vi "mock resonant image1.vi"() -> (0 "samples per period (var pix clock)":i32, 2 "var dwell time in ticks (2*pi)":i32[](graph) caption="dwell time in ticks (2*pi)", 3 "var dwell time in ticks (pi/2)":i16[](graph) caption="dwell time in ticks (pi/2)", 4 "samples per period (fix pix clock)":i32, 6 "fixed dwell time":i32)   [LabVIEW 2012]
uses:
  <vilib>/Analysis/NI_AALBase.lvlib
panel:
  out "avg dwell time":dbl
  out "x/y":dbl
  out "sum":i32
  out "cumsum 2":i32[](graph)
  in  "two lines per cycle":i32=2
  out "size(s)":i32
  out "samples per line":dbl
  out "cumsum":i32[](graph)
  out "Histogram Graph":T1(graph)
  in  "x pixels":i32=780
  out "Waveform Graph":dbl[](graph)
  out "Image":T2(plugin-control)
  in  "lines in y":i32=1
  in  "resonant frequency (eg. 8kHz)":i32=8000
  in  "sample clock (eg. 40 MHz)":i32=40000000
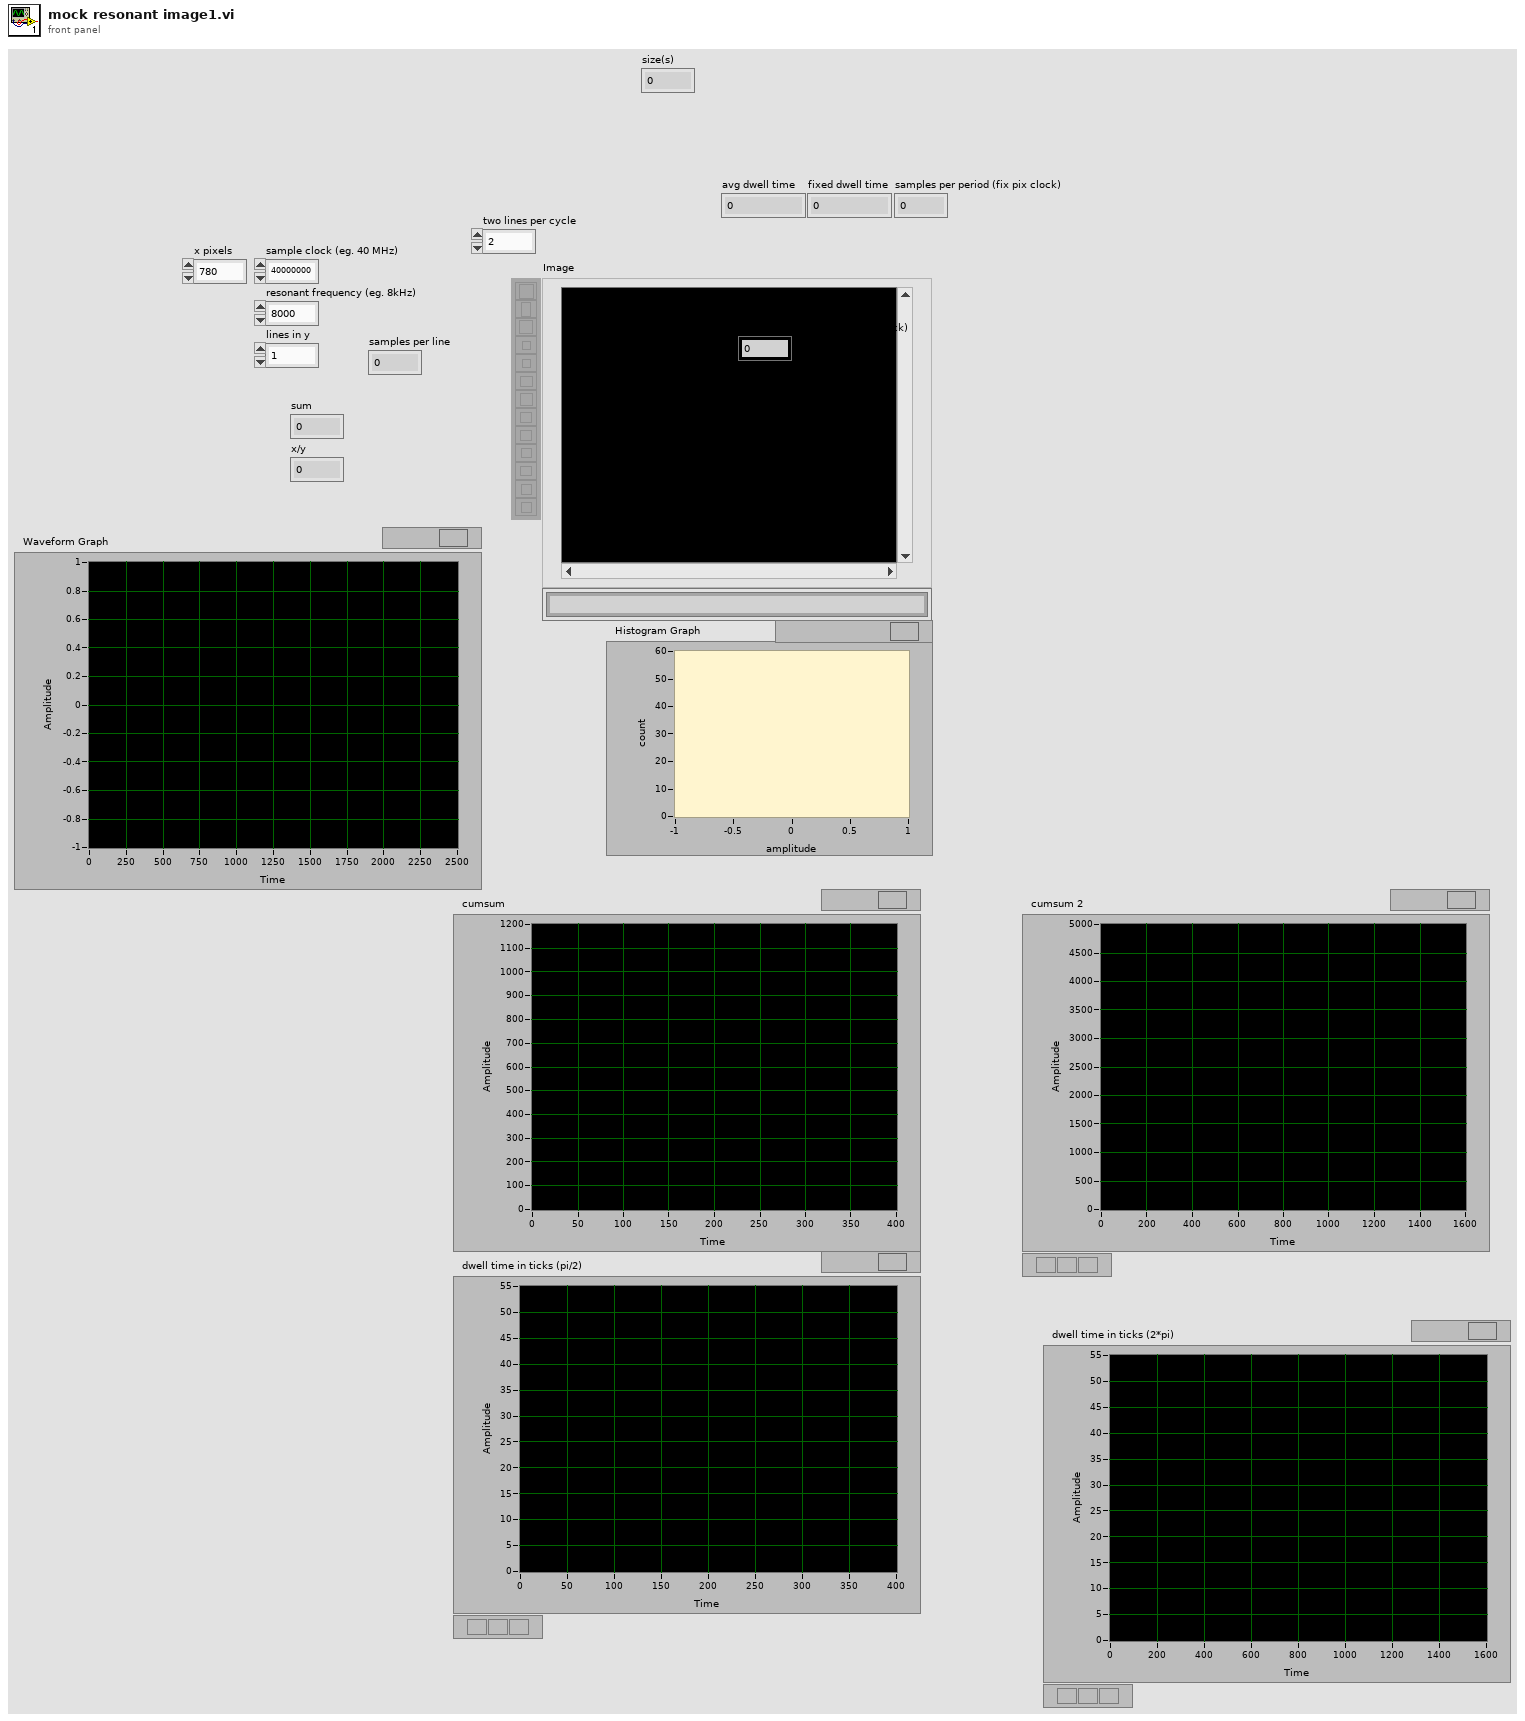
[diagram p1: front panel]
types:
  T1 = cluster{"X Values":dbl[], "Histogram: h(x)":i32[]}
  T2 = typedef "IMAQ Image.ctl" = refnum<image>
  T3 = typedef "Image Type" = u32
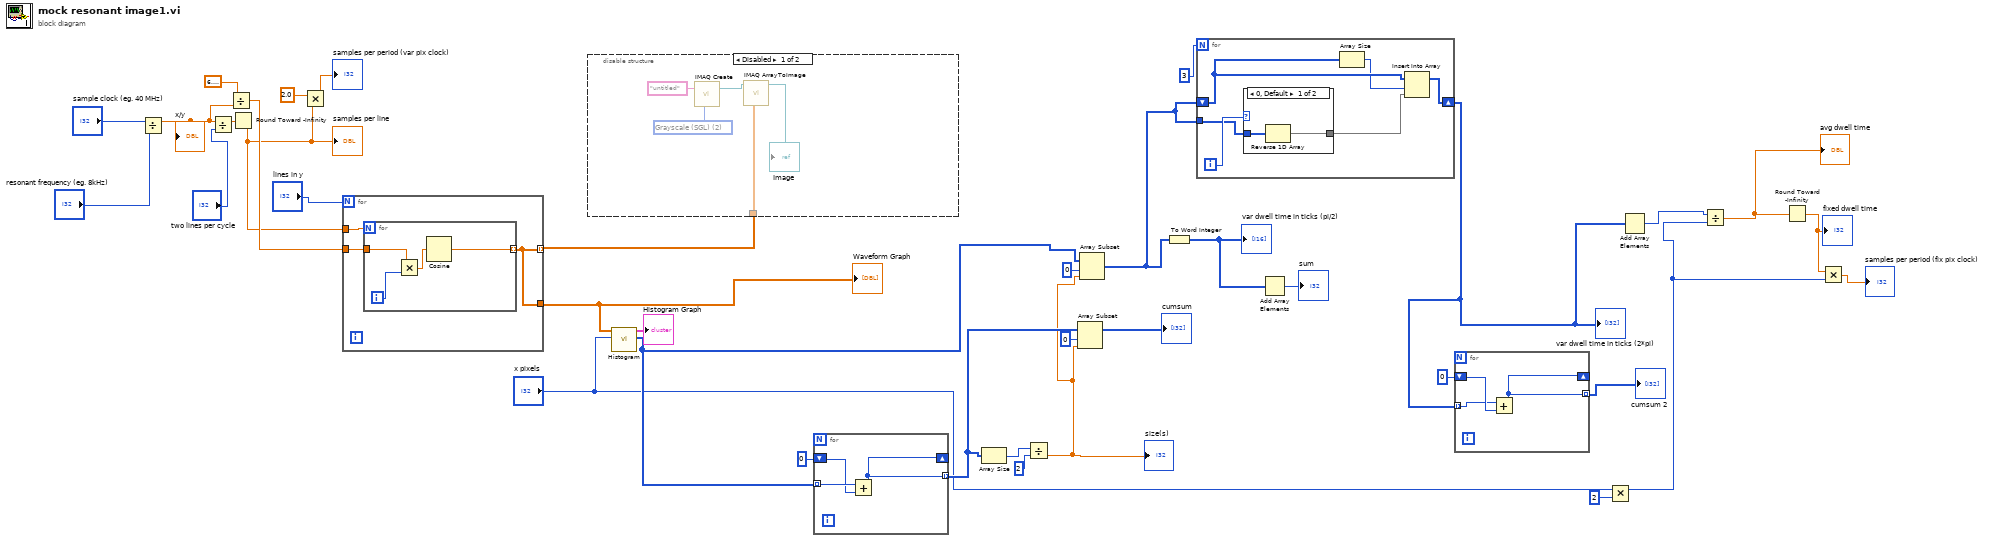
[diagram p0: block diagram]
diagram:
  n1 = Divide(x="sample clock (eg. 40 MHz)", y="resonant frequency (eg. 8kHz)") -> (x/y=w30:dbl)
  "x/y" <- w30
  n2 = Divide(x=w30, y="two lines per cycle") -> (x/y=w28:dbl)
  n3 = Divide(x=6.283185307179586, y=w30) -> (x/y=w35:dbl)
  n4 = Round Toward -Infinity(1:w28) -> (0:w3:dbl)
  "samples per line" <- w3
  n5 = Multiply(x=2.0, y=w3) -> (x*y=→"samples per period (var pix clock)":dbl)
  n6 = for {
    N: "lines in y" -> [_]
    tunnel: w3 -> [w40]
    tunnel: w35 -> [w39]
    tunnel: [w38] -> w33 mode=indexing
    tunnel: [w38] -> w32
    n7 = for {
      N: w40 -> [_]
      tunnel: w39 -> [w43]
      tunnel: [w41] -> w38 mode=indexing
      i -> [w42]
      n8 = Multiply(x=w43, y=w42) -> (x*y=w44:dbl)
      n9 = Cosine(x=w44) -> (cos(x)=w41:dbl)
    }
  }
  "Waveform Graph" <- w32
  n10 = disable-structure shown="Disabled" {
    disable-tunnel: w33 -> [w48 _]
    frame Disabled {
      w49 = T3 2 items=["Grayscale (U8)", "Grayscale (I16)", "Grayscale (SGL)", "Complex (CSG)", "RGB (U32)", "HSL (U32)", "RGB (U64)", "Grayscale (U16)"] ("Image Type")
      n11 = call "IMAQ Create"("Image Name"="untitled", "Image Type"=w49) -> ("New Image"=w47:T2)  [unwired: 3 in, 1 out]
      n12 = call "IMAQ ArrayToImage"("Image Pixels (Float)"=w48, "Image"=w47) -> ("Image Out"=→"Image":T2)  [unwired: 8 in, 1 out]
    }
    frame Enabled {
    }
  }
  n13 = call <vilib>:"Histogram.vi"("intervals"="x pixels", "X"=w32) -> ("Histogram: h(x)"=w20:i32[], "Histogram Graph"=→"Histogram Graph":T1)  [unwired: 6 in, 2 out]
  n14 = for {
    tunnel: w20 -> [w52] mode=indexing
    shift-right: [w50] -> _
    shift-left: 0 -> [w51]
    tunnel: [w50] -> w25 mode=indexing
    n15 = Add(x=w52, y=w51) -> (x+y=w50:i32)
  }
  n16 = Array Size(array=w25) -> (size(s)=w24:i32)
  n17 = Divide(x=w24, y=2 ("x")) -> (x/y=w19:dbl)
  "size(s)" <- w19
  n18 = Array Subset(array=w25, index=0, length=w19) -> (→"cumsum":i32[])
  n19 = Array Subset(array=w20, index=0, length=w19) -> (w14:i32[])
  n20 = To Word Integer(number=w14) -> (16bit integer=w12:i16[])
  "var dwell time in ticks (pi/2)" <- w12
  n21 = for {
    N: 3 -> [_]
    tunnel: w14 -> [w57]
    shift-right: [w53] -> w11
    shift-left: w14 -> [w56]
    i -> [w58]
    n22 = case shown="0, Default" w58 {
      tunnel: [w59 w61] -> w54
      tunnel: w57 -> [w60 w61]
      frame 0, Default {
        n23 = Reverse 1D Array(array=w60) -> (reversed array=w59:i32[])
      }
      frame 1 {
      }
    }
    n24 = Array Size(array=w56) -> (size(s)=w55:i32)
    n25 = Insert Into Array(array=w56, index=w55, new element=w54) -> (w53:i32[])
  }
  "var dwell time in ticks (2*pi)" <- w11
  n26 = Add Array Elements(numeric array=w12) -> (sum=→"sum":i16)
  n27 = for {
    shift-right: [w63] -> _
    shift-left: 0 -> [w64]
    tunnel: [w63] -> w15 mode=indexing
    tunnel: w11 -> [w62] mode=indexing
    n28 = Add(x=w62, y=w64) -> (x+y=w63:i32)
  }
  "cumsum 2" <- w15
  n29 = Multiply(x="x pixels", y=2) -> (x*y=w5:i32)
  n30 = Add Array Elements(numeric array=w11) -> (sum=w10:i32)
  n31 = Divide(x=w10, y=w5) -> (x/y=w9:dbl)
  "avg dwell time" <- w9
  n32 = Round Toward -Infinity(1:w9) -> (0:w8:dbl)
  "fixed dwell time" <- w8
  n33 = Multiply(x=w8, y=w5) -> (x*y=→"samples per period (fix pix clock)":dbl)
